vi "Counter Control.vi"   [LabVIEW 2020, in "BDAQ-6104.lvlib"]
uses:
  <instrlib>/BDAQ-6104/BDAQ-6104.lvlib
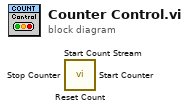
[diagram p0: block diagram]
diagram:
  n1 = call <instrlib>:"Reset Count.vi"() -> ()  [unwired: 10 in, 2 out]
  n2 = call <instrlib>:"Start Count Stream.vi"() -> ()  [unwired: 10 in, 2 out]
  n3 = call <instrlib>:"Stop Counter.vi"() -> ()  [unwired: 10 in, 2 out]
  n4 = call <instrlib>:"Start Counter.vi"() -> ()  [unwired: 10 in, 2 out]
